vi "KE622x -- Get Buf Readings Type.vi"(0 "Resource In":refnum<visa-resource-name>, 1 "Check For SCPI Errors? (T)":bool=TRUE, 11 "error in (no error)":errorcluster) -> (4 "Resource Out (dupl)":refnum<visa-resource-name>, 8 "Readings Type":T1, 15 "error out":errorcluster)   [LabVIEW 2010, in "Keithley 622x.lvlib"]
uses:
  Keithley 622x.lvlib
  Typedefs/KE622x -- Trace Buf Readings Type.ctl
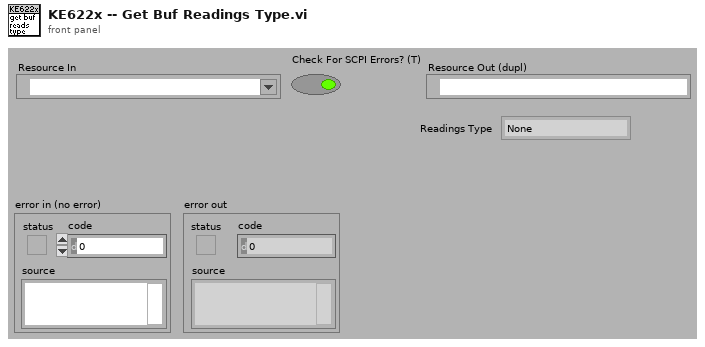
[diagram p1: front panel]
types:
  T1 = typedef "Keithley 622x.lvlib/KE622x -- Trace Buf Readings Type.ctl" = enum16{"None", "Delta", "Differential Cond", "Pulse Delta"}
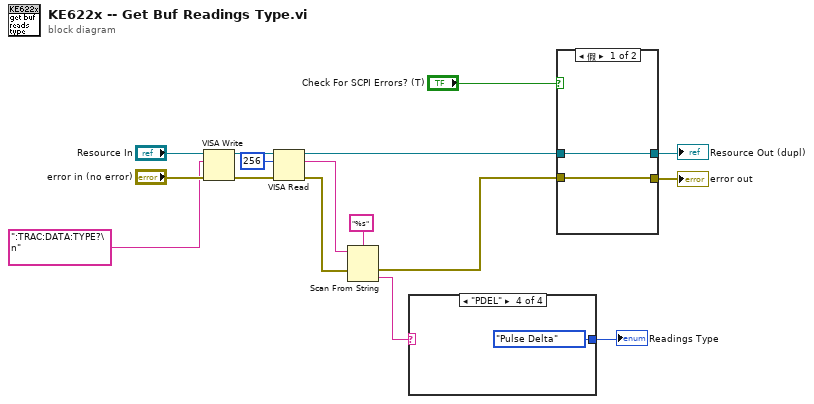
[diagram p0: block diagram]
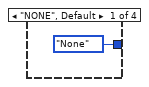
[diagram p2: hidden frame]
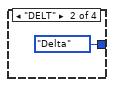
[diagram p3: hidden frame]
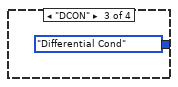
[diagram p4: hidden frame]
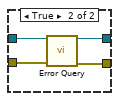
[diagram p5: hidden frame]
diagram:
  n1 = VISA Write(VISA resource name="Resource In", write buffer=":TRAC:DATA:TYPE?\n" ("format string"), error in (no error)="error in (no error)") -> (VISA resource name out=w10:refnum<visa-resource-name>, error out=w9:errorcluster)  [unwired: 1 out]
  n2 = VISA Read(VISA resource name=w10, byte count=u32 256, error in (no error)=w9) -> (VISA resource name out=w3:refnum<visa-resource-name>, read buffer=w5:string, error out=w7:errorcluster)  [unwired: 1 out]
  n3 = Scan From String(format string="%s", input string=w5, error in=w7) -> (error out=w4:errorcluster, output 1=w2:string)  [unwired: 2 in, 2 out]
  n4 = case shown="\"PDEL\"" w2 {
    tunnel: [KE622x_--_Trace_Buf_Readings_Type."None" ("Readings Type") KE622x_--_Trace_Buf_Readings_Type."Delta" ("Readings Type") KE622x_--_Trace_Buf_Readings_Type."Differential Cond" ("Readings Type") KE622x_--_Trace_Buf_Readings_Type."Pulse Delta" ("Readings Type")] -> w1
    frame "NONE", Default {
    }
    frame "DELT" {
    }
    frame "DCON" {
    }
    frame "PDEL" {
    }
  }
  "Readings Type" <- w1
  n5 = case shown="假" "Check For SCPI Errors? (T)" {
    tunnel: w3 -> [w22 w26]
    tunnel: w4 -> [w21 w25]
    tunnel: [w21 w24] -> w12
    tunnel: [w22 w23] -> w13
    frame False {
    }
    frame True {
      n6 = call "Error Query.vi"("VISA Resource In"=w26, "error in (no error)"=w25) -> ("VISA Resource Out (dupl)"=w23:refnum<visa-resource-name>, "error out"=w24:errorcluster)  [unwired: 10 in, 2 out]
    }
  }
  "Resource Out (dupl)" <- w13
  "error out" <- w12
